vi "PC_Puck_or_Player (DONE).vi"(8 "Error In":errorcluster, 10 "Cutoff":sgl, 11 "Circles Data":T1(array[cluster])) -> (0 "Error Out":errorcluster, 2 "Players":T2(array[cluster]), 3 "Puck":T2(array[cluster]))   [LabVIEW 2017]
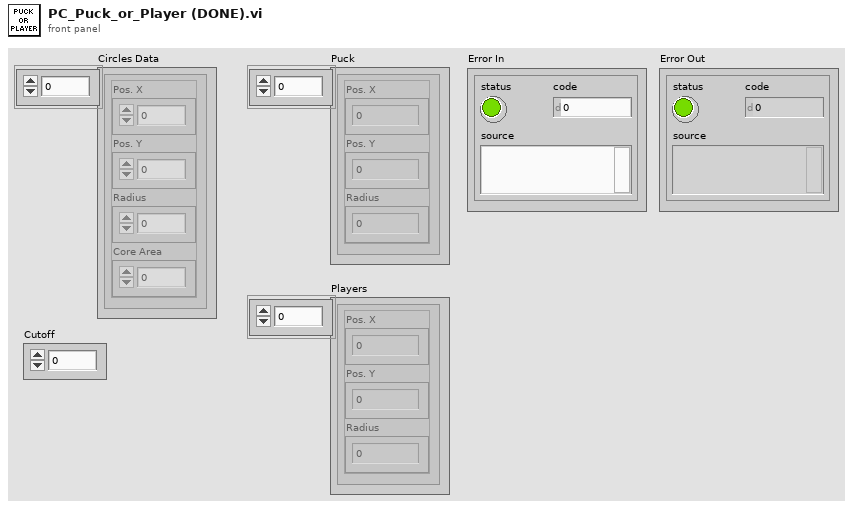
[diagram p1: front panel]
types:
  T1 = cluster{"Pos. X":i32, "Pos. Y":i32, "Radius":i32, "Core Area":i32}[]
  T2 = cluster{"Pos. X":i32, "Pos. Y":i32, "Radius":i32}[]
  T3 = cluster{"Pos. X":i32, "Pos. Y":i32, "Radius":i32}
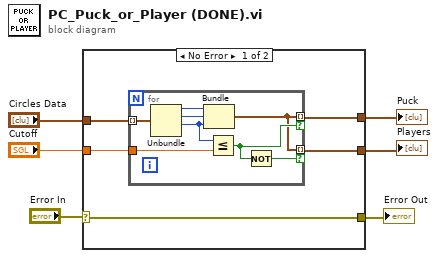
[diagram p0: block diagram]
diagram:
  n1 = case shown="No Error" "Error In" {
    selector: "Error In" -> [w7 w20]
    tunnel: [w11 _] -> w6
    tunnel: [w10 _] -> w5
    tunnel: "Cutoff" -> [w9 _]
    tunnel: "Circles Data" -> [w8 _]
    tunnel: [w7 w20] -> w1
    frame No Error {
      n2 = for {
        tunnel: w8 -> [w19] mode=indexing
        tunnel: w9 -> [w18]
        tunnel: [w13] -> w10 mode=indexing if=w14
        tunnel: [w13] -> w11 mode=indexing if=w12
        n3 = Unbundle(w19) -> ("Pos. X"=w17:i32, "Pos. Y"=w16:i32, "Radius"=w15:i32)  [unwired: 1 out]
        n4 = Bundle("Pos. X"=w17, "Pos. Y"=w16, "Radius"=w15) -> (w13:T3)  [unwired: 1 in]
        n5 = Less Or Equal?(x=w15, y=w18) -> (x <= y?=w14:bool)
        n6 = Not(x=w14) -> (.not. x?=w12:bool)
      }
    }
    frame Error {
    }
  }
  "Players" <- w6
  "Puck" <- w5
  "Error Out" <- w1
